vi "Handle Command.vi"(8 "error in (no error)":errorcluster, 9 "Data":variant, 10 "Command":string, 11 "instrument.PPMS2 in":refnum<class "instrument.PPMS2.lvclass">) -> (0 "error out":errorcluster, 1 "Processed Data":variant, 2 "Command":string, 3 "instrument.PPMS2 out":refnum<class "instrument.PPMS2.lvclass">)   [LabVIEW 2016, in "instrument.PPMS2.lvclass"]
uses:
  instrument.PPMS2.lvclass
  Typedefs/Temperature--PPMS2--cluster.ctl
  instrument.PPMS2.lvclass/instrument.PPMS2.ctl
  Typedefs/Magnet Field--PPMS2--cluster.ctl
  <userlib>/LevyLab/Levylab Instruments/Instrument Types/Cryostat/Typedefs/Magnet Mode--Enum.ctl
  Typedefs/Magnet Status--PPMS2--cluster.ctl
  Typedefs/Magnet Status--PPMS2--ring.ctl
  Typedefs/Temperature Status--PPMS2--cluster.ctl
  <userlib>/LevyLab/Levylab Instruments/Instrument Types/Cryostat/Instrument.Cryostat.lvclass
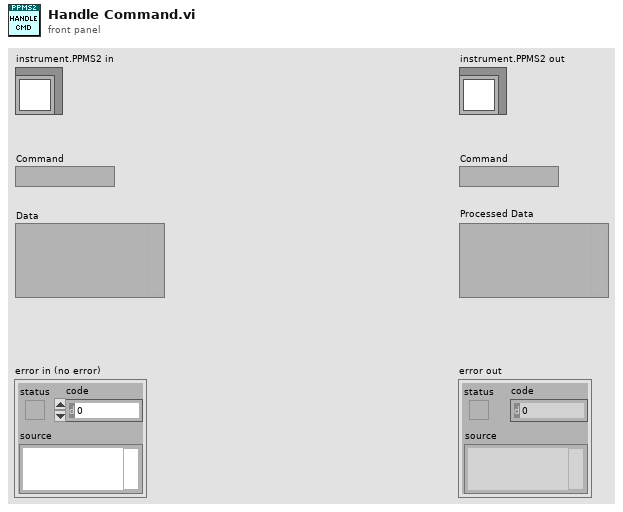
[diagram p1: front panel]
types:
  T1 = typedef "instrument.PPMS2.lvclass/Temperature--PPMS2--cluster.ctl" = cluster{"Temperature (K)":dbl, "Rate (K/min)":dbl}
  T2 = typedef "instrument.PPMS2.lvclass/Magnet Field--PPMS2--cluster.ctl" = cluster{"Target Field (Oe)":dbl, "Target Rate (Oe/s)":dbl, "Mode":T3}
  T3 = typedef "Instrument.Cryostat.lvclass/Magnet Mode--Enum.ctl" = enum16{"Persistent", "Driven"}
  T4 = enum16{"0", "1", "2", "3", "4", "5", "6", "7", "8", "9", "10", "11", "12", "13", "14"}
  T5 = typedef "instrument.PPMS2.lvclass/Magnet Status--PPMS2--cluster.ctl" = cluster{"Field (Oe)":dbl, "Field Status":T6}
  T6 = typedef "instrument.PPMS2.lvclass/Magnet Status--PPMS2--ring.ctl" = i32
  T7 = typedef "instrument.PPMS2.lvclass/Temperature Status--PPMS2--cluster.ctl" = cluster{"Temperature (K)":dbl, "Temperature Status":i32}
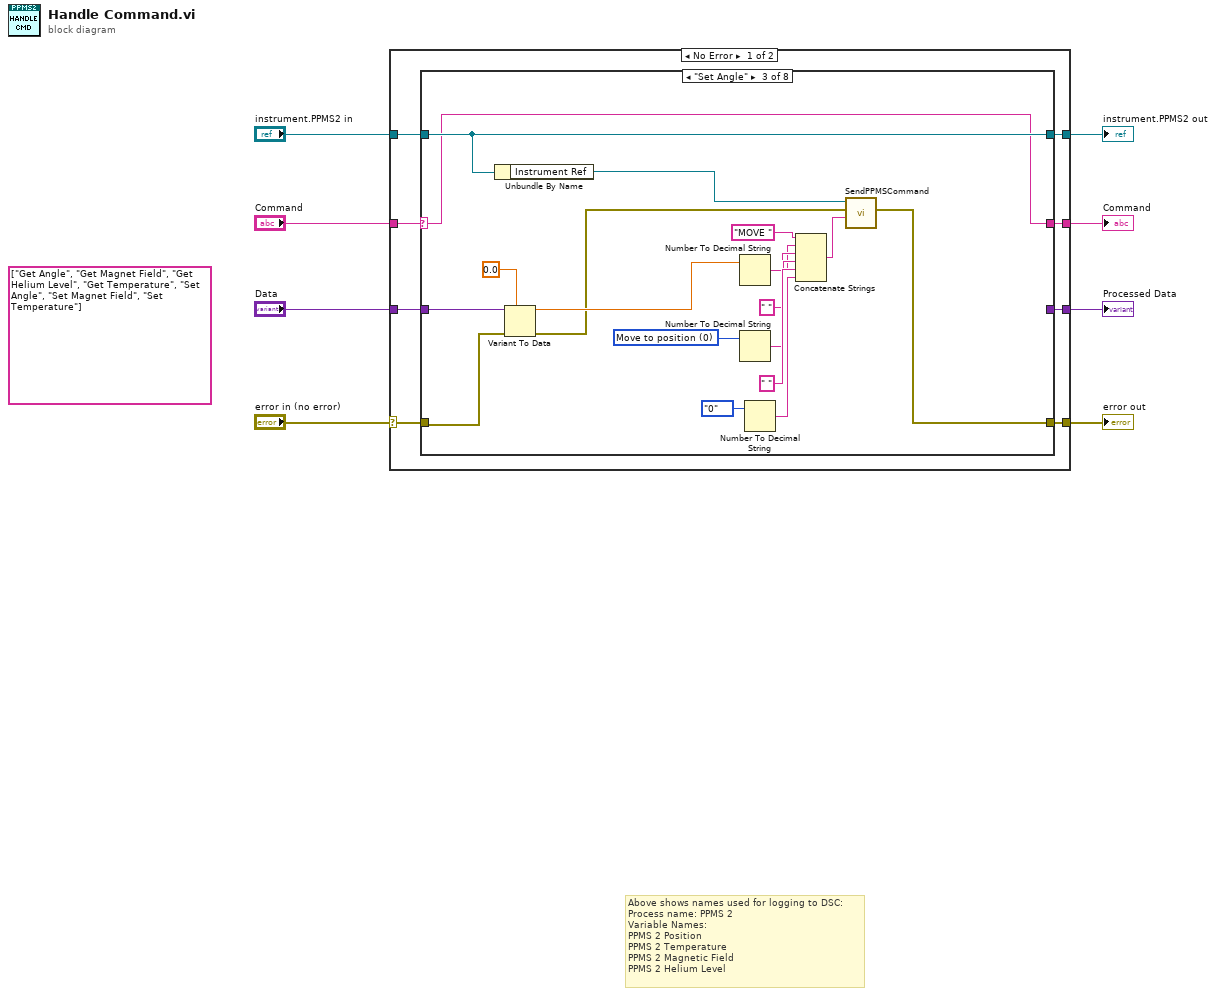
[diagram p0: block diagram]
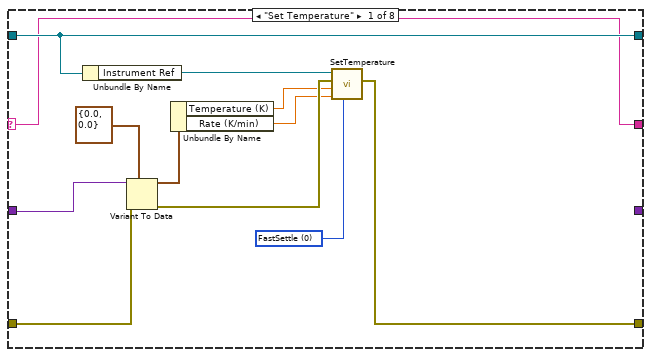
[diagram p2: hidden frame]
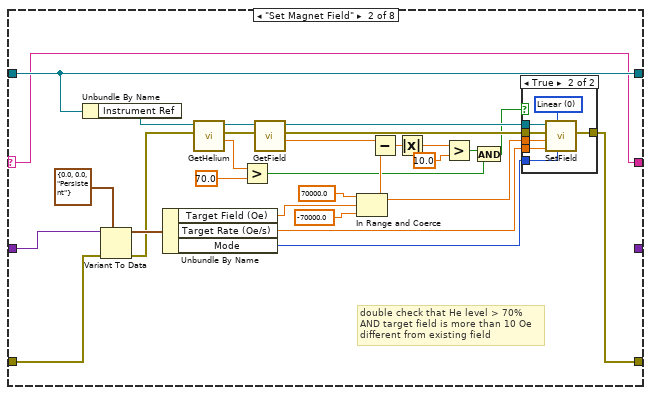
[diagram p3: hidden frame]
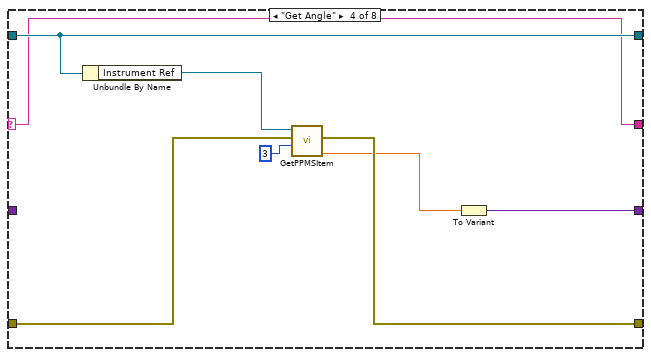
[diagram p5: hidden frame]
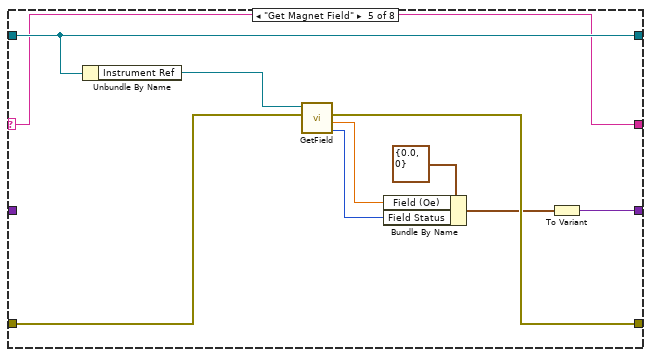
[diagram p6: hidden frame]
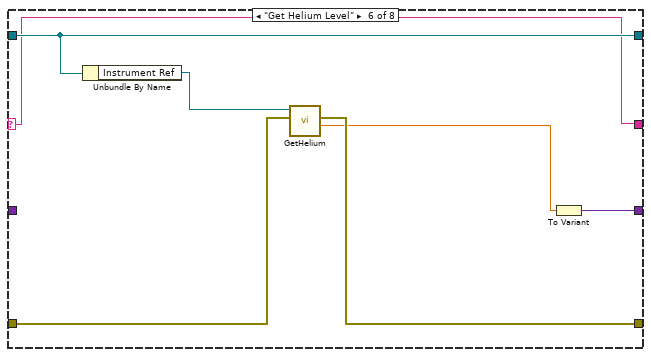
[diagram p7: hidden frame]
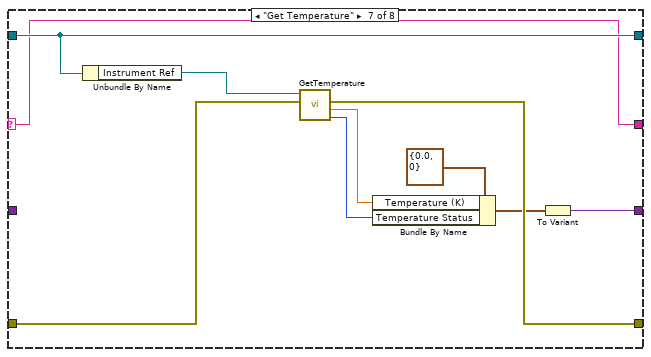
[diagram p8: hidden frame]
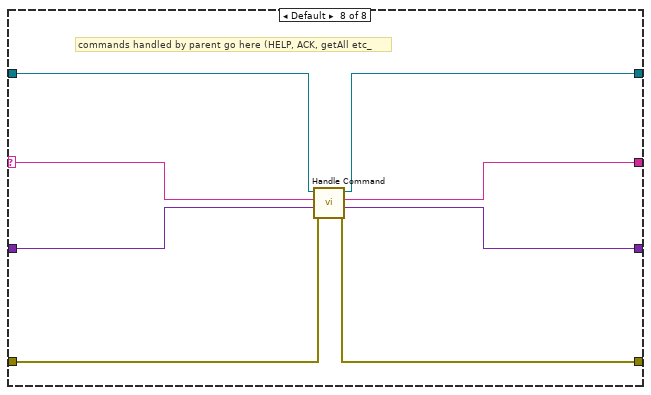
[diagram p9: hidden frame]
diagram:
  (unwired) string[] ["Get Angle", "Get Magnet Field", "Get Helium Level", "Get Temperature", "Set Angle", "Set Magnet Field", "Set Temperature"] ("Commands")
  # "Above shows names used for logging to DSC:\nProcess name: PPMS 2\nVariable Names:\nPPMS 2 Position\nPPMS 2 Temperature\nPPMS 2 Magnetic Field\nPPMS 2 Helium Level"
  n1 = case shown="No Error" "error in (no error)" {
    selector: "error in (no error)" -> [w11 w126]
    tunnel: [w10 w126] -> w6
    tunnel: [w16 _] -> w4
    tunnel: [w15 _] -> w5
    tunnel: [w14 w127] -> w7
    tunnel: "Data" -> [w13 _]
    tunnel: "Command" -> [w9 _]
    tunnel: "instrument.PPMS2 in" -> [w12 w127]
    frame No Error {
      n2 = case shown="\"Set Angle\"" w9 {
        selector: w9 -> [w17 w29 w65 w83 w91 w101 w108 w118]
        tunnel: [_ _ _ w84 w92 w103 w113 w125] -> w16
        tunnel: [w17 w29 w65 w83 w91 w101 w108 w124] -> w15
        tunnel: [w28 w56 w82 w90 w100 w107 w117 w123] -> w14
        tunnel: w13 -> [w23 w54 w70 _ _ _ _ w122]
        tunnel: w12 -> [w28 w56 w82 w90 w100 w107 w117 w121]
        tunnel: w11 -> [w25 w53 w71 w87 w98 w106 w115 w120]
        tunnel: [w26 w51 w66 w86 w97 w105 w114 w119] -> w10
        frame "Set Temperature" {
          w18 = 0 items=["FastSettle", "NoOvershoot"] ("Approach")
          n3 = Unbundle By Name(w28) -> ("Instrument Ref"=w27:refnum<k24>)
          n4 = Variant To Data(error in=w25, type=T1 {"Temperature (K)"=0.0, "Rate (K/min)"=0.0} ("Temperature"), Variant=w23) -> (data=w22:T1, error out=w21:errorcluster)
          n5 = Unbundle By Name(w22) -> ("Temperature (K)"=w20:dbl, "Rate (K/min)"=w19:dbl)
          n6 = call "SetTemperature.vi"("Approach"=w18, "Rate"=w19, "Temperature"=w20, "error in (no error)"=w21, "Instrument Ref In"=w27) -> ("error out"=w26:errorcluster)  [unwired: 2 in, 2 out]
        }
        frame "Set Magnet Field" {
          # "double check that He level > 70%\nAND target field is more than 10 Oe\ndifferent from existing field"
          n7 = Unbundle By Name(w56) -> ("Instrument Ref"=w37:refnum<k24>)
          n8 = Variant To Data(error in=w53, type=T2 {"Target Field (Oe)"=0.0, "Target Rate (Oe/s)"=0.0, "Mode"=enum."Persistent"} ("Magnet Field"), Variant=w54) -> (data=w52:T2, error out=w50:errorcluster)
          n9 = Unbundle By Name(w52) -> ("Target Field (Oe)"=w40:dbl, "Target Rate (Oe/s)"=w43:dbl, "Mode"=w31:T3)
          n10 = call "GetHelium.vi"("error in (no error)"=w50, "Instrument Refnum in"=w37) -> ("Helium Level (%)"=w44:dbl, "error out"=w49:errorcluster, "Instrument Ref Out"=w47:refnum<k24>)  [unwired: 3 in]
          n11 = Greater?(x=w44, y=70.0) -> (0:w32:bool)
          n12 = call "GetField.vi"("error in (no error)"=w49, "Instrument Ref In"=w47) -> ("Field"=w35:dbl, "error out"=w48:errorcluster, "Instrument Ref Out"=w46:refnum<k24>)  [unwired: 3 in, 2 out]
          n13 = In Range and Coerce(upper limit=70000.0, x=w40, lower limit=-70000.0) -> (coerced(x)=w36:dbl)  [unwired: 1 out]
          n14 = Subtract(x=w35, y=w36) -> (x-y=w34:dbl)
          n15 = Absolute Value(x=w34) -> (abs(x)=w39:dbl)
          n16 = Greater?(x=w39, y=10.0) -> (0:w33:bool)
          n17 = And(x=w33, y=w32) -> (x .and. y?=w30:bool)
          n18 = case shown="True" w30 {
            tunnel: [w57 w63] -> w51
            tunnel: w48 -> [w57 w62]
            tunnel: w46 -> [_ w61]
            tunnel: w43 -> [_ w60]
            tunnel: w36 -> [_ w59]
            tunnel: w31 -> [_ w58]
            frame False {
            }
            frame True {
              w64 = 0 items=["Linear", "NoOvershoot", "Oscillate"] ("Approach")
              n19 = call "SetField.vi"("Mode"=w58, "Approach"=w64, "Rate"=w60, "Field"=w59, "error in (no error)"=w62, "Instrument Ref In"=w61) -> ("error out"=w63:errorcluster)  [unwired: 1 in, 2 out]
            }
          }
        }
        frame "Set Angle" {
          w76 = u16 0 items=["Move to position", "Move to limit", "Redefine current position", ""] ("Mode")
          n20 = Unbundle By Name(w82) -> ("Instrument Ref"=w72:refnum<k24>)
          n21 = Variant To Data(error in=w71, type=0.0 ("Target Position"), Variant=w70) -> (data=w68:dbl, error out=w67:errorcluster)
          n22 = Number To Decimal String(number=w68) -> (decimal integer string=w74:string)  [unwired: 1 in]
          n23 = Number To Decimal String(number=w76) -> (decimal integer string=w77:string)  [unwired: 1 in]
          n24 = Number To Decimal String(number=T4."0" ("Slow down code\ndefault = 0")) -> (decimal integer string=w80:string)  [unwired: 1 in]
          n25 = Concatenate Strings("MOVE " ("string"), w74, " " ("string"), w77, " " ("string"), w80) -> (w81:string)
          n26 = call "SendPPMSCommand.vi"("PpmsCommand"=w81, "error in (no error)"=w67, "Instrument Ref In"=w72) -> ("error out"=w66:errorcluster)  [unwired: 4 in, 4 out]
        }
        frame "Get Angle" {
          n27 = Unbundle By Name(w90) -> ("Instrument Ref"=w88:refnum<k24>)
          n28 = call "GetPPMSItem.vi"("Channel"=3, "error in (no error)"=w87, "Instrument Ref In"=w88) -> ("Result"=w85:dbl, "error out"=w86:errorcluster)  [unwired: 1 in, 2 out]
          n29 = To Variant(anything=w85) -> (Variant=w84:variant)
        }
        frame "Get Magnet Field" {
          n30 = Unbundle By Name(w100) -> ("Instrument Ref"=w99:refnum<k24>)
          n31 = call "GetField.vi"("error in (no error)"=w98, "Instrument Ref In"=w99) -> ("Field\nStatus"=w95:i32, "Field"=w96:dbl, "error out"=w97:errorcluster)  [unwired: 3 in, 2 out]
          n32 = Bundle By Name(cluster=T5 {"Field (Oe)"=0.0, "Field Status"=0}, "Field (Oe)"=w96, "Field Status"=w95) -> (w93:T5)
          n33 = To Variant(anything=w93) -> (Variant=w92:variant)
        }
        frame "Get Helium Level" {
          n34 = Unbundle By Name(w107) -> ("Instrument Ref"=w102:refnum<k24>)
          n35 = call "GetHelium.vi"("error in (no error)"=w106, "Instrument Refnum in"=w102) -> ("Helium Level (%)"=w104:dbl, "error out"=w105:errorcluster)  [unwired: 3 in, 1 out]
          n36 = To Variant(anything=w104) -> (Variant=w103:variant)
        }
        frame "Get Temperature" {
          n37 = Unbundle By Name(w117) -> ("Instrument Ref"=w116:refnum<k24>)
          n38 = call "GetTemperature.vi"("error in (no error)"=w115, "Instrument Ref In"=w116) -> ("Temperature\nStatus"=w111:i32, "Temperature"=w112:dbl, "error out"=w114:errorcluster)  [unwired: 3 in, 2 out]
          n39 = Bundle By Name(cluster=T7 {"Temperature (K)"=0.0, "Temperature Status"=0}, "Temperature (K)"=w112, "Temperature Status"=w111) -> (w109:T7)
          n40 = To Variant(anything=w109) -> (Variant=w113:variant)
        }
        frame Default {
          # "commands handled by parent go here (HELP, ACK, getAll etc_"
          n41 = call-parent "Handle Command.vi"("error in (no error)"=w120, "Data"=w122, "Command"=w118, "Instrument in"=w121) -> ("error out"=w119:errorcluster, "Processed Data"=w125:variant, "Command"=w124:string, "Instrument out"=w123:refnum<class "instrument.PPMS2.lvclass">)  [unwired: 4 in]
        }
      }
    }
    frame Error {
    }
  }
  "error out" <- w6
  "instrument.PPMS2 out" <- w7
  "Processed Data" <- w4
  "Command" <- w5
